vi "CreateScanFilename.vi"() -> ()   [LabVIEW 2013]
uses:
  controls/Microprobe Vars.ctl
  controls/ProgramColumn.ctl
panel:
  out "Sample name":string
  in  "Current row":string[](array[string])
  in  "Probe Target State":T1 {"Tset" format="%.1f"; "Telem" format="%.1f"; "GasC" format="%.1g"; "GasB" format="%.1f"; "GasA" format="%.1f"; "Z" format="%.3g"; "Y" format="%.3g"; "X" format="%.3g"; "RampRate" format="%.1f"}
  in  "Sample directory":path
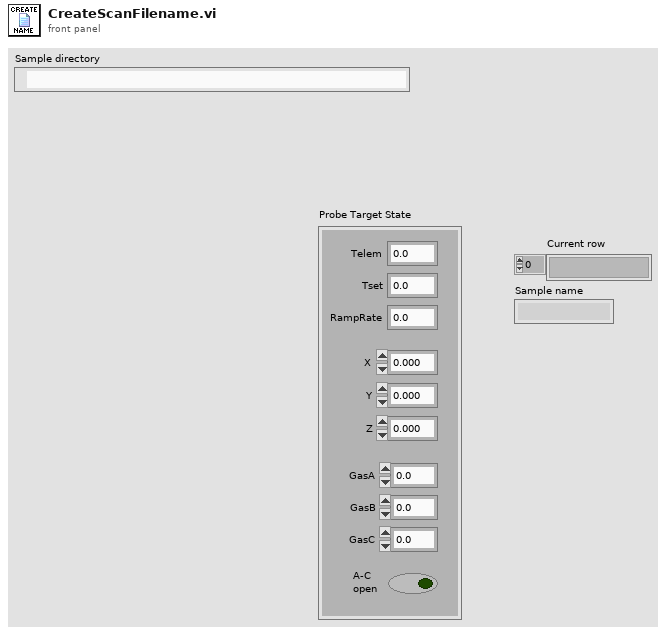
[diagram p1: front panel]
types:
  T1 = typedef "Microprobe Vars.ctl" = cluster{"Telem":dbl, "Tset":dbl, "RampRate":dbl, "X":dbl, "Y":dbl, "Z":dbl, "GasA":dbl, "GasB":dbl, "GasC":dbl, "A-C\nopen":bool}
  T2 = typedef "ProgramColumn.ctl" = enum16{"Run Number", "Stage Temperature", "Ramp Rate", "Gas A", "Gas B", "Gas C", "Row index I", "Column index J", "X position", "Y position", "Z position", "Voltage", "Highest frequency", "Lowest frequency", "Number of freq pts"}
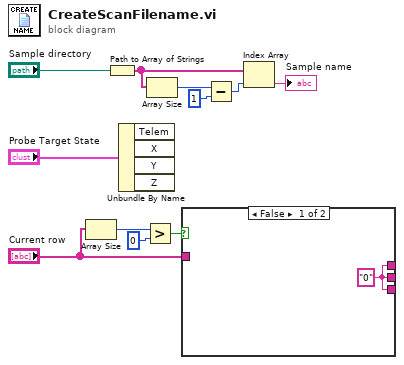
[diagram p0: block diagram]
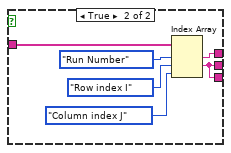
[diagram p2: hidden frame]
diagram:
  n1 = Array Size(array="Current row") -> (size(s)=w4:i32)
  n2 = Path to Array of Strings(0:"Sample directory") -> (2:w10:string[])  [unwired: 1 out]
  n3 = Unbundle By Name("Probe Target State") -> ()  [unwired: 4 out]
  n4 = Greater?(x=w4, y=0) -> (0:w2:bool)
  n5 = Array Size(array=w10) -> (size(s)=w9:i32)
  n6 = case shown="False" w2 {
    tunnel: "Current row" -> [_ w15]
    tunnel: [w12 w14] -> _
    tunnel: [w12 w13] -> _
    tunnel: [w12 w13] -> _
    frame False {
      w12 = "0"
    }
    frame True {
      n7 = Index Array(array=w15, index #1=ProgramColumn."Run Number" ("Enum"), index #2=ProgramColumn."Row index I" ("Enum"), index #3=ProgramColumn."Column index J" ("Enum")) -> (element #1=w14:string, element #2=w13:string)  [unwired: 1 out]
    }
  }
  n8 = Subtract(x=w9, y=1) -> (x-y=w8:i32)
  n9 = Index Array(array=w10, index=w8) -> (element=→"Sample name":string)
